vi "settings.vi"(11 "Test Mode":T1(radio)) -> ()   [LabVIEW 2014]
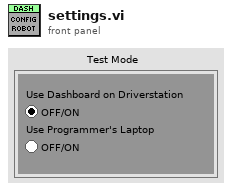
[diagram p1: front panel]
types:
  T1 = enum32{"Use Dashboard on Driverstation", "Use Programmer's Laptop"}
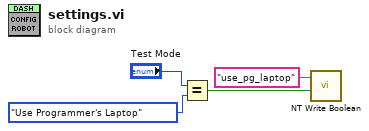
[diagram p0: block diagram]
diagram:
  n1 = Equal?(x="Test Mode", y=T1."Use Programmer's Laptop") -> (x = y?=w2:bool)
  n2 = call <vilib>:"NT Write Boolean.vi"("Boolean"=w2, "Name"="use_pg_laptop") -> ()  [unwired: 9 in, 1 out]
